vi "fgv_DynamicEvent_measureTool.vi"(7 "Event FGV Actions":T1, 8 "error in (no error)":errorcluster, 10 "event data":string="FGV Event") -> (0 "error out":errorcluster, 2 "Event Registration Refnum":refnum<event-registration>, 3 "element":refnum<user-event>)   [LabVIEW 2020]
doc: "Functional Global Variable which can register and store a reference to a Dynamic User Event. Main VI with an Event Structure must first to register the event before the 'Fire Event' case can be used. Otherwise, an error is returned."
uses:
  Event FGV Actions.ctl
panel:
  # "Input"
  # "Output"
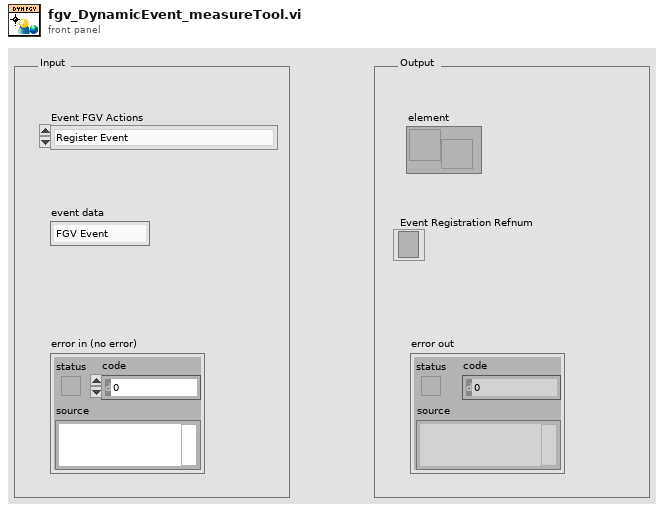
[diagram p1: front panel]
types:
  T1 = typedef "Event FGV Actions.ctl" = enum16{"Register Event", "Fire Event", "Release Event"}
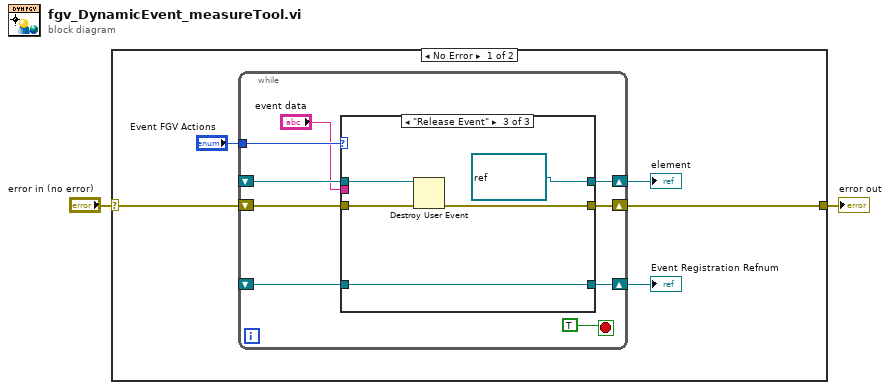
[diagram p0: block diagram]
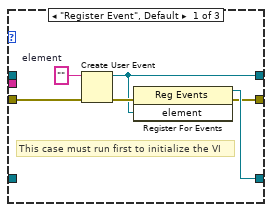
[diagram p2: hidden frame]
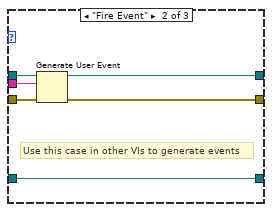
[diagram p3: hidden frame]
diagram:
  n1 = case shown="No Error" "error in (no error)" {
    selector: "error in (no error)" -> [w6 w34]
    tunnel: [w5 w34] -> w1
    frame No Error {
      n2 = while {
        tunnel: "Event FGV Actions" -> [w15]
        shift-right: [w13] -> w3
        shift-left: _ -> [w9]
        shift-right: [w14] -> w4
        shift-left: _ -> [w12]
        shift-right: [w10] -> w5
        shift-left: w6 -> [w11]
        stop <- TRUE stop-if-true
        n3 = case shown="\"Release Event\"" w15 {
          tunnel: [w20 w26 refnum<user-event> refnum ("user event")] -> w14
          tunnel: [w19 w24 w29] -> w13
          tunnel: w12 -> [_ w28 w31]
          tunnel: w11 -> [w18 w27 w33]
          tunnel: [w17 w25 w32] -> w10
          tunnel: w9 -> [_ w24 w29]
          tunnel: "event data" -> [_ w23 _]
          frame "Register Event", Default {
            w21 = ""  # element
            # "This case must run first to initialize the VI"
            n4 = Create User Event(user event datatype=w21, error in=w18) -> (user event=w20:refnum<user-event>, error out=w22:errorcluster)
            n5 = register-events(error in=w22, w20) -> (reference out=w19:refnum<event-registration>, error out=w17:errorcluster)  [unwired: 1 in]
          }
          frame "Fire Event" {
            # "Use this case in other VIs to generate events"
            n6 = Generate User Event(user event=w28, event data cluster=w23, error in=w27) -> (user event out=w26:refnum<user-event>, error out=w25:errorcluster)  [unwired: 1 in]
          }
          frame "Release Event" {
            n7 = Destroy User Event(user event=w31, error in=w33) -> (error out=w32:errorcluster)
          }
        }
      }
      "element" <- w4
      "Event Registration Refnum" <- w3
    }
    frame Error {
    }
  }
  "error out" <- w1
